vi "PositionerCapture_HoloLoader.vi"() -> ()   [LabVIEW 2011]
doc: "CONEX - CC Virtual Front Panel:\n\nThis is a sample of an application that can be built with the LabVIEW drivers.\n\nPress HOME / ENABLE in top left of panel to put stage in Ready state for motion."
uses:
  <vilib>/userDefined/High Color/IMAQdx.ctl
  C:/Users/Lab541/Desktop/David_Maluenda MAIN FOLDER/System/SupportFiles/Control 1.ctl
  <vilib>/Platform/TimedLoop/XDataNode/timing_clust.ctl
  <vilib>/Platform/TimedLoop/XDataNode/nitl_modes.ctl
  <vilib>/Platform/TimedLoop/XDataNode/wakeup.ctl
  <vilib>/Platform/TimedLoop/XDataNode/XDataNode.xnode
  <vilib>/Platform/TimedLoop/XDataNode/XDNodeRunTimeDep.lvlib
  <vilib>/vision/driver/NI_Vision_Acquisition_Software.lvlib
  <vilib>/vision/NI_Vision_Development_Module.lvlib
panel:
  in  "Units":T1 caption="nm" items=["mm", "um", "nm", "lam"]
  out "test":path
  in  "Session In":T2="BW14bits Paraxial"
  in  "stop":bool
  out "Slide":u8(slide) scale=0.0..100.0
  out "# Sat. Pixels":sgl(slide) scale=1.0..800000.0
  out "Unsatured":bool
  out "pathY":path
  out "pathX":path
  in  "Xoffset1 2":dbl=-1300.0
  out "X position 3":dbl
  in  "Fine: 3":dbl(slide)=8.165680473372781 scale=0.0..10.0
  in  "X position 2":dbl(slide)=3.78698224852071 scale=0.0..10.0
  in  "Yoffset1 2":dbl=-150.0
  out "Y position 2":dbl
  in  "Fine:":dbl(slide)=1.694915254237288 scale=0.0..10.0
  in  "Y position 2":dbl(slide)=1.9318181818181817 scale=0.0..10.0
  in  "Yoffset1":dbl=-300.0
  in  "Xoffset1":dbl=1300.0
  out "Y position 1":dbl
  out "X position":dbl
  in  "Fine:":dbl(slide)=3.8983050847457625 scale=0.0..10.0
  in  "Fine:":dbl(slide)=5.502958579881657 scale=0.0..10.0
  in  "Y position":dbl(slide)=3.5028248587570623 scale=0.0..10.0
  in  "X position 1":dbl(slide)=3.4319526627218933 scale=0.0..10.0
  out "String 4":string
  out "CGHy":T3(plugin-control)
  out "CGHx":T3(plugin-control)
  out "path":path
  in  "Holo:":dbl=1.0
  out "Current noUnits":dbl caption="mm" format="%#_6f"
  in  "lambda":dbl caption="nm" format="%#_6f"
  in  "Units":string(combo)="mm"
  in  "Go0":bool
  in  "Zero position":dbl caption="lam" format="%#_6f"
  in  "Tare":bool
  out "Relative position":dbl caption="lam" format="%#_6f"
  in  "Path to save the captures":path
  out "Image":T3(plugin-control)
  in  "(1) Go to:":dbl=1.0 caption="lam"
  out "Title":string
  in  "Set Max":bool
  in  "Set Min":bool
  in  "Max":dbl
  in  "Min":dbl
  in  "Set velocity":bool
  out "Stop cycle":bool=TRUE
  out "Title 2":string
  in  "Cycle":bool
  in  "Go2":bool
  in  "Go1":bool
  in  "(2) Go to:":dbl=1.0 caption="lam"
  in  "-":bool
  in  "+":bool
  in  "Step:":dbl caption="lam" format="%#_6f"
  out "Position History":dbl(graph)=1.5
  in  "Action":bool
  out "Stop polling":bool=TRUE
  out "Controller state description":string="STATUS"
  out "Velocity MAX":dbl=0.4
  out "Controller state":string="33"
  out "Positioner error":string="0000"
  in  "Velocity:":dbl format="%#_6f"
  in  "Exit":bool=TRUE
  out "Target position":dbl
  in  "Exit":bool
  in  "Position glissière":cluster{dbl, dbl}(slide) scale=0.0..25.0
  out "Current position":dbl caption="lam" format="%#_6f"
  # "mm/s"
  # "mm"
  # "Limits:"
  # "mm"
  # "(1)"
  # "(2)"
  # "%"
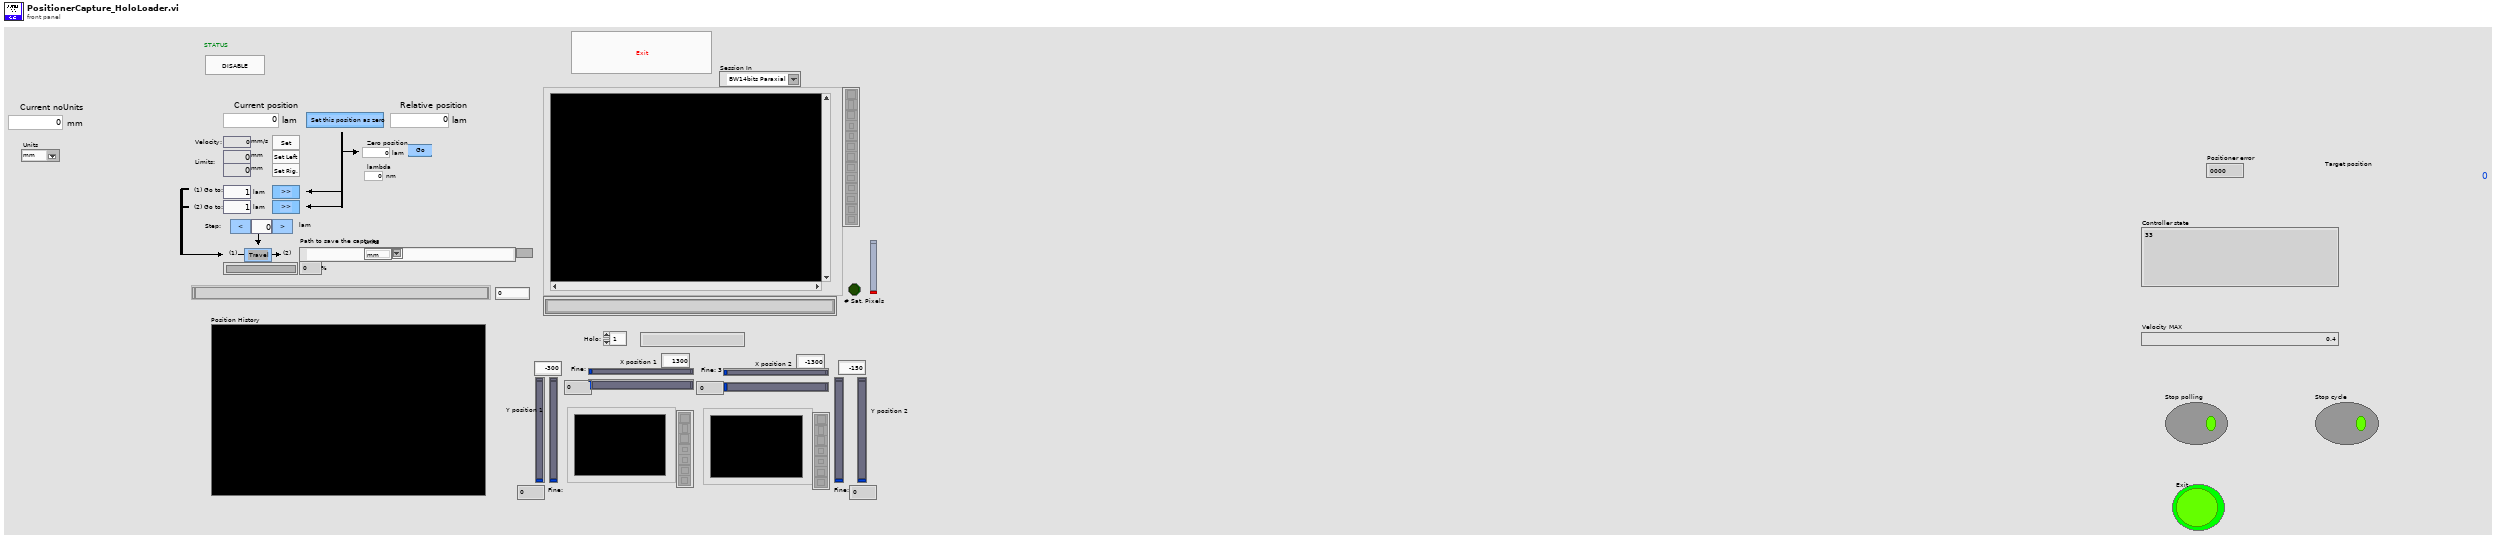
[diagram p1: front panel]
types:
  T1 = typedef "Control 1.ctl" = dbl
  T2 = typedef "IMAQdx.ctl" = refnum<k21>
  T3 = typedef "IMAQ Image.ctl" = refnum<image>
  T4 = enum8{"Enabled", "Disabled", "Disabled and Grayed Out"}
  T5 = typedef "XDNodeRunTimeDep.lvlib/timing_clust.ctl" = cluster{"Expected End [f-1]":u64, "Actual End [f-1]":u64, "Finished Late? [f-1]":bool, "Expected End [i-1]":u64, "Actual End [i-1]":u64, "Finished Late? [i-1]":bool, "Expected Start [i]":u64, "Actual Start [i]":u64, "Expected Start [f]":u64, "Actual Start [f]":u64, "Source Name":string, "Structure Name":string, "Period":i64, "Deadline":i64, "Offset":i64, "Start":i64, "Priority":i32, "Timeout":i32, "Mode":T6, "Wakeup Reason":T7, "Error":errorcluster, "Source Type":string, "Secondary Source Type":string, "Global End Time":u64, "Global Start Time":u64, "Frame Duration":u64, "Iteration Duration":u64, "Assigned CPU":i32, "I/O Scan Engine Mode":u32}
  T6 = typedef "XDNodeRunTimeDep.lvlib/nitl_modes.ctl" = enum32{"No Change", "Process missed periods, maintain original phase", "Discard missed periods, maintain original phase", "Process missed periods, ignore original phase", "Discard missed periods, ignore original phase"}
  T7 = typedef "XDNodeRunTimeDep.lvlib/wakeup.ctl" = enum32{"Normal", "Aborted", "Asynchronous wakeup", "Timing source error", "Timed loop error", "Timeout"}
  T8 = cluster{"VISA resource name":refnum<visa-resource-name>, "Device name":string, "Controller address":i32, "error":errorcluster}
  T9 = cluster{"Starting Value":sgl, "Incremental Value":sgl, "Histogram":u32[]}
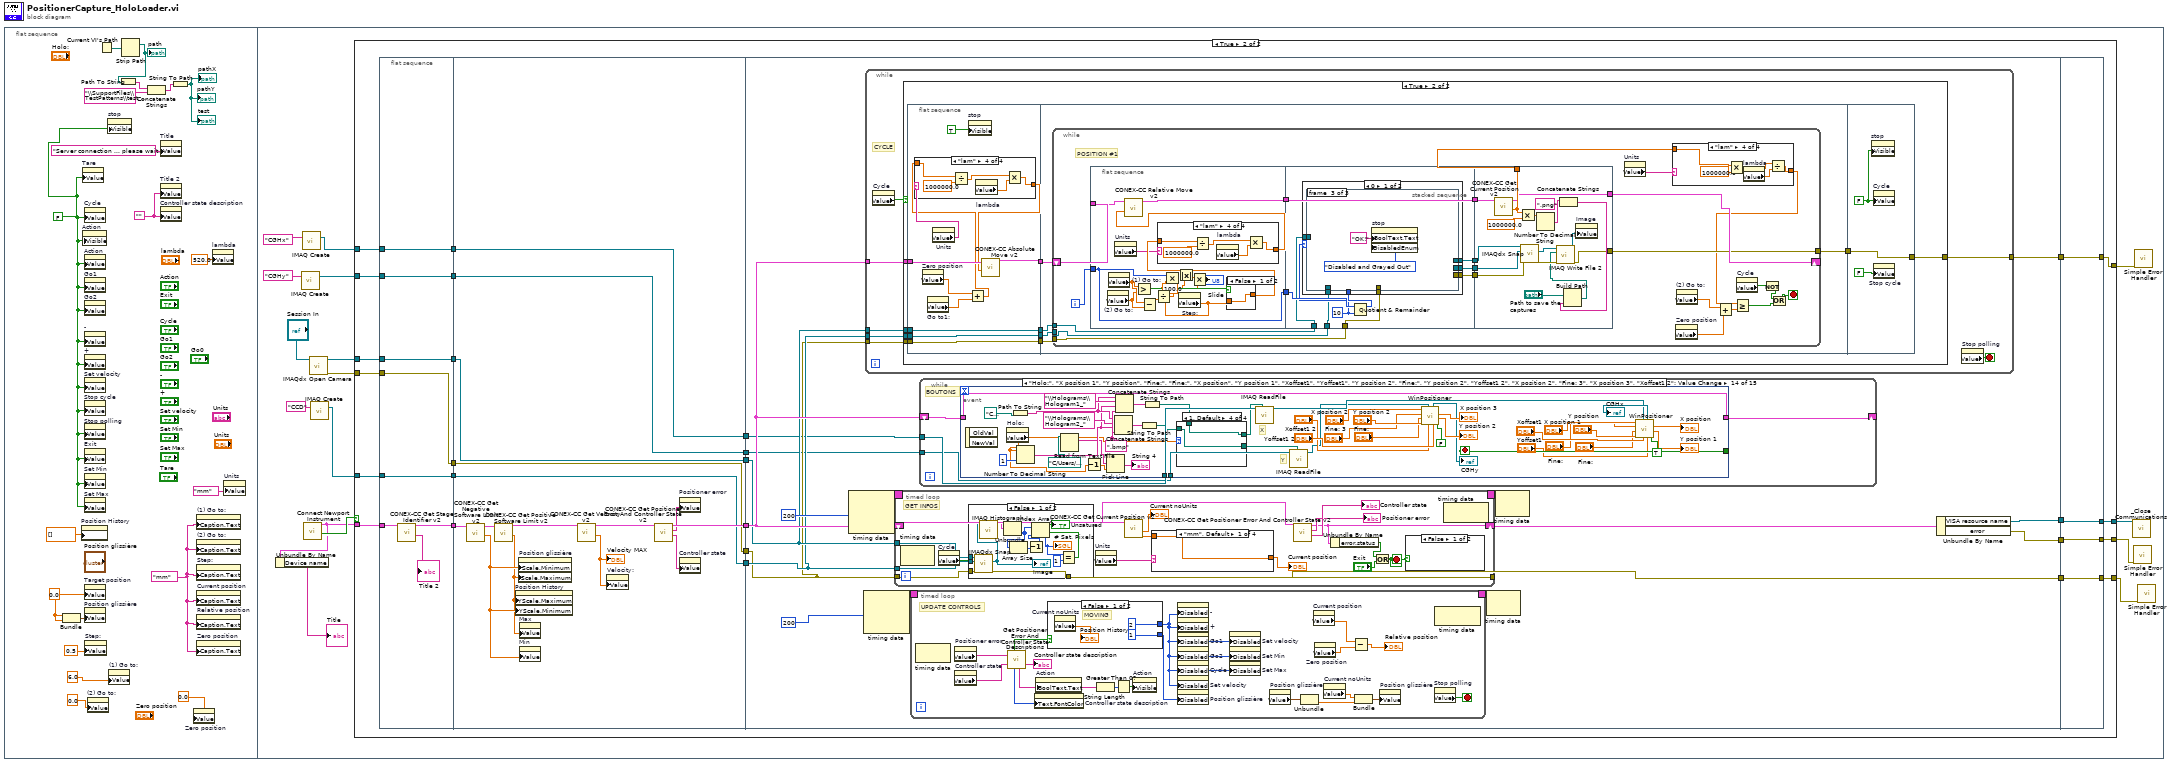
[diagram p0: block diagram]
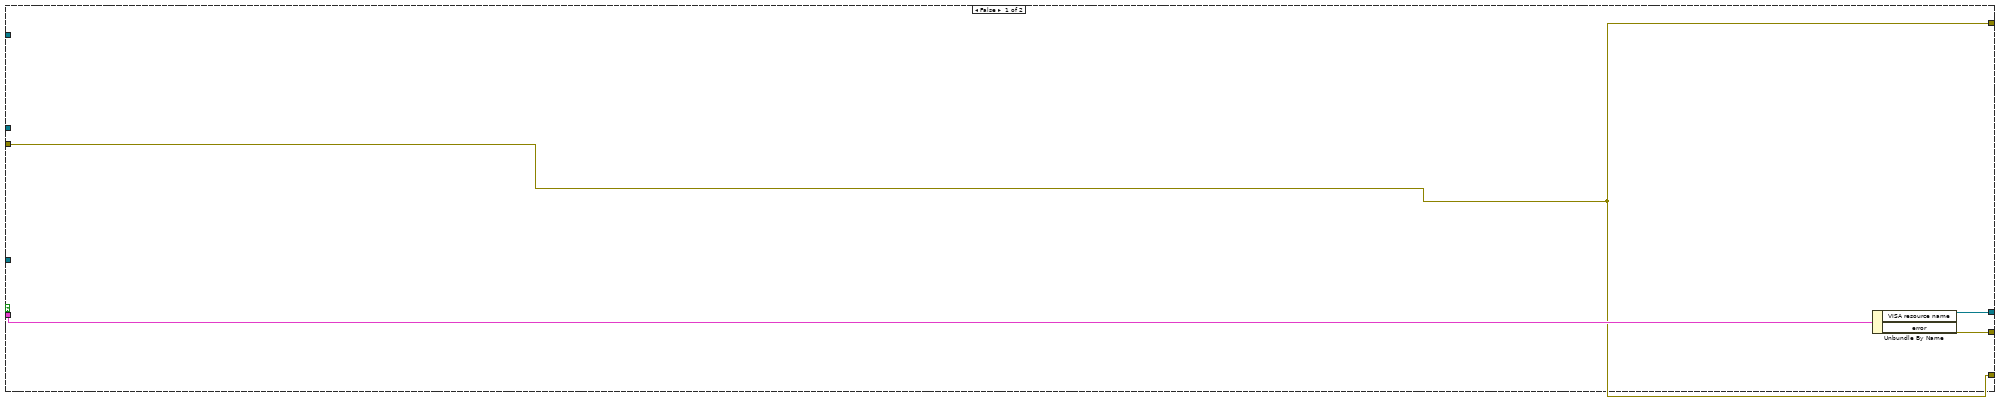
[diagram p2: hidden frame]
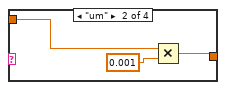
[diagram p5: hidden frame]
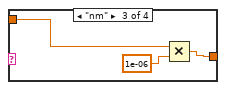
[diagram p6: hidden frame]
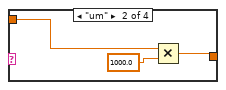
[diagram p8: hidden frame]
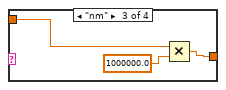
[diagram p9: hidden frame]
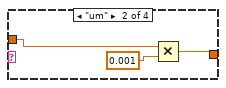
[diagram p11: hidden frame]
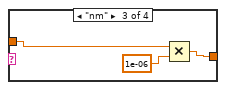
[diagram p12: hidden frame]
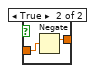
[diagram p13: hidden frame]
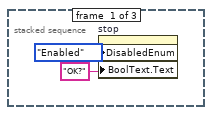
[diagram p14: hidden frame]
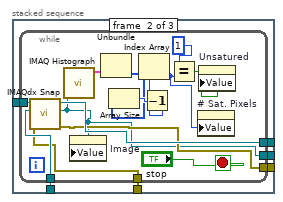
[diagram p15: hidden frame]
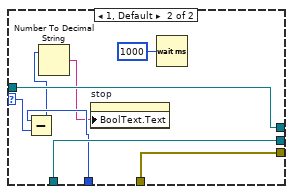
[diagram p16: hidden frame]
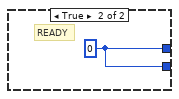
[diagram p17: hidden frame]
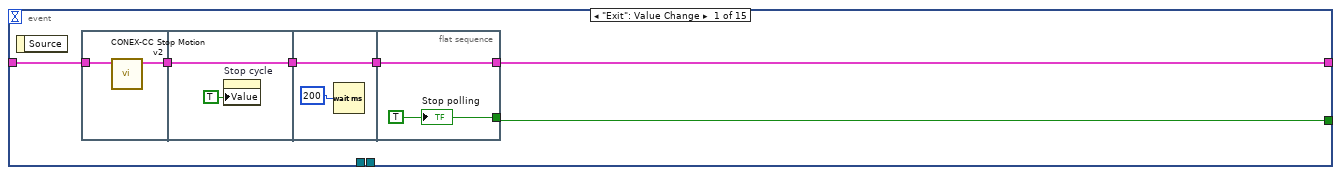
[diagram p18: hidden frame]
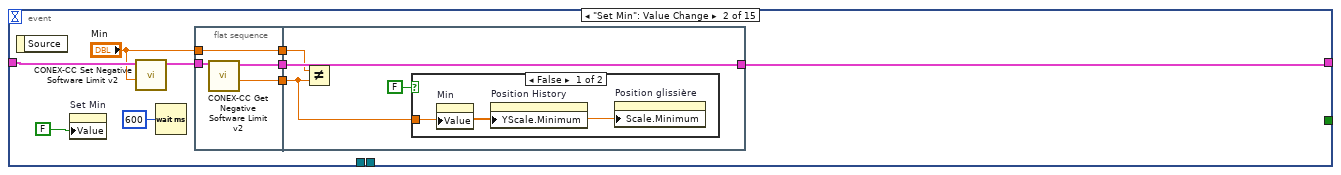
[diagram p19: hidden frame]
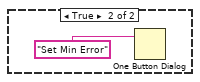
[diagram p20: hidden frame]
diagram:
  n1 = flat-sequence {
    frame #0 {
      w9 = "mm" ("Units")
      w1 = FALSE
      w18 = 0.0
      w17 = ""
      n2 = Bundle(w18, w18) -> (w19:cluster{dbl, dbl})  [unwired: 1 out]
      n3 = property on="Position History" class="WFChart (strict)"("History Data"=dbl[] [] ("Données d'historique")) -> ()  [unwired: 2 in, 2 out]
      n4 = property on="Tare" class="Bool (strict)"("Value"=w1) -> ()  [unwired: 2 in, 2 out]
      n5 = property on="Action" class="Bool (strict)"("Visible"=w1) -> ()  [unwired: 2 in, 2 out]
      n6 = property on="Cycle" class="Bool (strict)"("Value"=w1) -> ()  [unwired: 2 in, 2 out]
      n7 = property on="Action" class="Bool (strict)"("Value"=w1) -> ()  [unwired: 2 in, 2 out]
      n8 = property on="Go1" class="Bool (strict)"("Value"=w1) -> ()  [unwired: 2 in, 2 out]
      n9 = property on="Go2" class="Bool (strict)"("Value"=w1) -> ()  [unwired: 2 in, 2 out]
      n10 = property on="-" class="Bool (strict)"("Value"=w1) -> ()  [unwired: 2 in, 2 out]
      n11 = property on="+" class="Bool (strict)"("Value"=w1) -> ()  [unwired: 2 in, 2 out]
      n12 = property on="Set velocity" class="Bool (strict)"("Value"=w1) -> ()  [unwired: 2 in, 2 out]
      n13 = property on="Stop cycle" class="Bool (strict)"("Value"=w1) -> ()  [unwired: 2 in, 2 out]
      n14 = property on="Stop polling" class="Bool (strict)"("Value"=w1) -> ()  [unwired: 2 in, 2 out]
      n15 = property on="Exit" class="Bool (strict)"("Value"=w1) -> ()  [unwired: 2 in, 2 out]
      n16 = property on="Set Min" class="Bool (strict)"("Value"=w1) -> ()  [unwired: 2 in, 2 out]
      n17 = property on="Set Max" class="Bool (strict)"("Value"=w1) -> ()  [unwired: 2 in, 2 out]
      n18 = property on="Target position" class="DigNum (strict)"("Value"=w18) -> ()  [unwired: 2 in, 2 out]
      n19 = property on="Position glissière" class="Slide (strict)"("Value"=w19) -> ()  [unwired: 2 in, 2 out]
      n20 = property on="Step:" class="DigNum (strict)"("Value"=0.5 ("Step")) -> ()  [unwired: 2 in, 2 out]
      n21 = property on="(2) Go to:" class="DigNum (strict)"("Value"=0.0 ("Abs. Move 2")) -> ()  [unwired: 2 in, 2 out]
      n22 = Current VI's Path() -> (path=w7:path)
      n23 = property on="stop" class="Bool"("Visible"=w1) -> ()  [unwired: 2 in, 2 out]
      n24 = property on="(1) Go to:" class="DigNum (strict)"("Value"=6.0 ("Abs. Move 1")) -> ()  [unwired: 2 in, 2 out]
      n25 = Strip Path(path=w7) -> (stripped path=w6:path)  [unwired: 1 out]
      "path" <- w6
      n26 = Path To String(path=w6) -> (string=w5:string)
      n27 = Concatenate Strings(w5, "\\SupportFiles\\TestPatterns\\test_pattern.bmp" ("string")) -> (w3:string)
      n28 = property on="Title" class="Str"("Value"="Server connection ... please wait." ("Title")) -> ()  [unwired: 2 in, 2 out]
      n29 = property on="Title 2" class="Str"("Value"=w17) -> ()  [unwired: 2 in, 2 out]
      n30 = property on="Controller state description" class="Str"("Value"=w17) -> ()  [unwired: 2 in, 2 out]
      n31 = String To Path(string=w3) -> (path=→"pathX" →"pathY" →"test":path)
      n32 = property on="Zero position" class="DigNum (strict)"("Value"=0.0 ("Zero position")) -> ()  [unwired: 2 in, 2 out]
      n33 = property on="(1) Go to:" class="DigNum (strict)"("Caption.Text"=w9) -> ()  [unwired: 2 in, 2 out]
      n34 = property on="(2) Go to:" class="DigNum (strict)"("Caption.Text"=w9) -> ()  [unwired: 2 in, 2 out]
      n35 = property on="Step:" class="DigNum (strict)"("Caption.Text"=w9) -> ()  [unwired: 2 in, 2 out]
      n36 = property on="Current position" class="DigNum (strict)"("Caption.Text"=w9) -> ()  [unwired: 2 in, 2 out]
      n37 = property on="Relative position" class="DigNum (strict)"("Caption.Text"=w9) -> ()  [unwired: 2 in, 2 out]
      n38 = property on="Zero position" class="DigNum (strict)"("Caption.Text"=w9) -> ()  [unwired: 2 in, 2 out]
      n39 = property on="lambda" class="DigNum (strict)"("Value"=520.0 ("lambda")) -> ()  [unwired: 2 in, 2 out]
      n40 = property on="Units" class="CmbBox"("Value"="mm" ("Units")) -> ()  [unwired: 2 in, 2 out]
    }
    frame #1 {
      n41 = call "IMAQ Create"("Image Name"="CGHy") -> ("New Image"=w21:T3)  [unwired: 4 in, 1 out]
      n42 = call "IMAQ Create"("Image Name"="CGHx") -> ("New Image"=w20:T3)  [unwired: 4 in, 1 out]
      n43 = call <userlib>:"Connect Newport Instrument.vi"() -> ("Connected"=w33:bool, "Device Connection Cluster"=w32:T8)  [unwired: 7 in, 3 out]
      n44 = Unbundle By Name(w32) -> ("Device name"=→"Title":string)
      n45 = call <vilib>:"IMAQdx Open Camera.vi"("Session In"="Session In") -> ("error out"=w26:errorcluster, "Session Out"=w28:T2)  [unwired: 9 in]
      n46 = call "IMAQ Create"("Image Name"="CCD") -> ("New Image"=w27:T3)  [unwired: 4 in, 1 out]
      n47 = case shown="True" w33 {
        tunnel: [w38 w65] -> w35
        tunnel: w32 -> [w39 w63]
        tunnel: [w37 w59] -> w31
        tunnel: w28 -> [_ w57]
        tunnel: w27 -> [_ w54]
        tunnel: w26 -> [w36 w51]
        tunnel: [w36 w48] -> w25
        tunnel: [w36 w46] -> w24
        tunnel: w21 -> [_ w44]
        tunnel: w20 -> [_ w41]
        frame False {
          n48 = Unbundle By Name(w39) -> ("VISA resource name"=w37:refnum<visa-resource-name>, "error"=w38:errorcluster)
        }
        frame True {
          n49 = flat-sequence {
            tunnel: w63 -> [w73]
            tunnel: [w71] -> w62
            tunnel: [w70] -> w58
            tunnel: w57 -> [w70]
            tunnel: [w69] -> w55
            tunnel: w54 -> [w69]
            tunnel: [w68] -> w52
            tunnel: w51 -> [w68]
            tunnel: [w67] -> w45
            tunnel: w44 -> [w67]
            tunnel: [w66] -> w42
            tunnel: w41 -> [w66]
            tunnel: [w85] -> w64
            tunnel: w62 -> [w82]
            tunnel: w58 -> [w78]
            tunnel: [w78] -> w56
            tunnel: w55 -> [w77]
            tunnel: [w77] -> w53
            tunnel: w52 -> [w76]
            tunnel: [w76] -> w50
            tunnel: w45 -> [w75]
            tunnel: [w75] -> w43
            tunnel: w42 -> [w74]
            tunnel: [w74] -> w40
            tunnel: w64 -> [w96]
            tunnel: [w98] -> w61
            tunnel: [w97] -> w60
            tunnel: w56 -> [w95]
            tunnel: w53 -> [w94]
            tunnel: w50 -> [w93]
            tunnel: [w92] -> w49
            tunnel: [w91] -> w47
            tunnel: w43 -> [w90]
            tunnel: w40 -> [w89]
            tunnel: [w616] -> w65
            tunnel: w61 -> [w615]
            tunnel: w60 -> [w616]
            tunnel: [w615] -> w59
            tunnel: [w614] -> w48
            tunnel: w49 -> [w614]
            tunnel: [w613] -> w46
            tunnel: w47 -> [w613]
            frame #0 {
              n50 = call <userlib>:"CONEX-CC Get Stage Identifier v2.vi"("Connection Cluster in"=w73) -> ("Identifier"=→"Title 2":string, "Connection Cluster out"=w71:T8)  [unwired: 9 in]
            }
            frame #1 {
              n51 = call <userlib>:"CONEX-CC Get Negative Software Limit v2.vi"("Connection Cluster in"=w82) -> ("Left limit"=w87:dbl, "Connection Cluster out"=w81:T8)  [unwired: 9 in]
              n52 = call <userlib>:"CONEX-CC Get Positive Software Limit v2.vi"("Connection Cluster in"=w81) -> ("Right limit"=w86:dbl, "Connection Cluster out"=w80:T8)  [unwired: 9 in]
              n53 = property on="Position History" class="WFChart (strict)"("YScale.Maximum"=w86, "YScale.Minimum"=w87) -> ()  [unwired: 2 in, 2 out]
              n54 = property on="Position glissière" class="Slide (strict)"("Scale.Minimum"=w87, "Scale.Maximum"=w86) -> ()  [unwired: 2 in, 2 out]
              n55 = property on="Max" class="DigNum (strict)"("Value"=w86) -> ()  [unwired: 2 in, 2 out]
              n56 = property on="Min" class="DigNum (strict)"("Value"=w87) -> ()  [unwired: 2 in, 2 out]
              n57 = call <userlib>:"CONEX-CC Get Velocity v2.vi"("Connection Cluster in"=w80) -> ("Velocity"=w88:dbl, "Connection Cluster out"=w79:T8)  [unwired: 8 in, 1 out]
              "Velocity MAX" <- w88
              n58 = property on="Velocity:" class="DigNum (strict)"("Value"=w88) -> ()  [unwired: 2 in, 2 out]
              n59 = call <userlib>:"CONEX-CC Get Positioner Error And Controller State v2.vi"("Connection Cluster in"=w79) -> ("Controller state"=w83:string, "Positioner error"=w84:string, "Connection Cluster out"=w85:T8)  [unwired: 8 in]
              n60 = property on="Positioner error" class="Str"("Value"=w84) -> ()  [unwired: 2 in, 2 out]
              n61 = property on="Controller state" class="Str"("Value"=w83) -> ()  [unwired: 2 in, 2 out]
            }
            frame #2 {
              n62 = node-c288(i64 200 ("Période")) -> (w105:T5)  [unwired: 1 in, 1 out]
              n63 = node-c288(i64 200 ("Période")) -> (w103:T5)  [unwired: 1 in, 1 out]
              n64 = while {
                tunnel: w96 -> [w112]
                tunnel: w95 -> [w109]
                tunnel: w94 -> [w108]
                tunnel: w93 -> [w107]
                tunnel: [w106] -> w91
                stop <- w111 stop-if-true
                # "CYCLE"
                n65 = property on="Cycle" class="Bool (strict)"() -> ("Value"=w110:bool)  [unwired: 2 in, 2 out]
                n66 = case shown="True" w110 {
                  tunnel: w112 -> [_ w123]
                  tunnel: w109 -> [_ w120]
                  tunnel: w108 -> [_ w118]
                  tunnel: w107 -> [w113 w116]
                  tunnel: [w113 w115] -> w106
                  frame False {
                  }
                  frame True {
                    n67 = flat-sequence {
                      tunnel: w123 -> [w134]
                      tunnel: [w133] -> w122
                      tunnel: [w132] -> w121
                      tunnel: w120 -> [w132]
                      tunnel: [w131] -> w119
                      tunnel: w118 -> [w131]
                      tunnel: [w130] -> w117
                      tunnel: w116 -> [w130]
                      tunnel: w122 -> [w151]
                      tunnel: w121 -> [w150]
                      tunnel: w119 -> [w149]
                      tunnel: w117 -> [w148]
                      tunnel: [w147] -> w114
                      tunnel: [w284] -> w115
                      tunnel: w114 -> [w284]
                      frame #0 {
                        n68 = property on="Zero position" class="DigNum (strict)"() -> ("Value"=w125:dbl)  [unwired: 2 in, 2 out]
                        n69 = property on="Go to1:" class="DigNum (strict)"() -> ("Value"=w127:dbl)  [unwired: 2 in, 2 out]
                        n70 = property on="Units" class="CmbBox"() -> ("Value"=w128:string)  [unwired: 2 in, 2 out]
                        n71 = property on="stop" class="Bool"("Visible"=TRUE) -> ()  [unwired: 2 in, 2 out]
                        n72 = Add(x=w125, y=w127) -> (x+y=w126:dbl)
                        n73 = case shown="\"lam\"" w128 {
                          tunnel: [w135 w136 w139 w142] -> w129
                          tunnel: w126 -> [w135 w137 w140 w146]
                          frame "mm", Default {
                          }
                          frame "um" {
                            n74 = Multiply(x=w137, y=0.001) -> (x*y=w136:dbl)
                          }
                          frame "nm" {
                            n75 = Multiply(x=w140, y=1e-06) -> (x*y=w139:dbl)
                          }
                          frame "lam" {
                            n76 = Divide(x=w146, y=1000000.0) -> (x/y=w144:dbl)
                            n77 = property on="lambda" class="DigNum (strict)"() -> ("Value"=w143:dbl)  [unwired: 2 in, 2 out]
                            n78 = Multiply(x=w144, y=w143) -> (x*y=w142:dbl)
                          }
                        }
                        n79 = call <userlib>:"CONEX-CC Absolute Move v2.vi"("Target position"=w129, "Connection Cluster in"=w134) -> ("Connection Cluster out"=w133:T8)  [unwired: 5 in, 2 out]
                      }
                      frame #1 {
                        n80 = while {
                          shift-right: [w173] -> _
                          shift-left: w151 -> [w174]
                          tunnel: w150 -> [w163]
                          tunnel: w149 -> [w162]
                          tunnel: w148 -> [w161]
                          tunnel: [w172] -> w147
                          i -> [w160]
                          stop <- w159 stop-if-true
                          # "POSITION #1"
                          n81 = flat-sequence {
                            tunnel: w174 -> [w202]
                            tunnel: [w201] -> w166
                            tunnel: w160 -> [w187]
                            tunnel: [w187] -> w155
                            tunnel: w166 -> [w227]
                            tunnel: [w227] -> w165
                            tunnel: w163 -> [w224]
                            tunnel: w162 -> [w223]
                            tunnel: w161 -> [w222]
                            tunnel: w155 -> [w226]
                            tunnel: [w221] -> w154
                            tunnel: [w220] -> w153
                            tunnel: [w219] -> w152
                            tunnel: w165 -> [w279]
                            tunnel: [w271] -> w171
                            tunnel: [w270] -> w173
                            tunnel: [w269] -> w172
                            tunnel: w154 -> [w268]
                            tunnel: w153 -> [w267]
                            tunnel: w152 -> [w266]
                            frame #0 {
                              n82 = property on="(2) Go to:" class="DigNum (strict)"() -> ("Value"=w194:dbl)  [unwired: 2 in, 2 out]
                              n83 = property on="(1) Go to:" class="DigNum (strict)"() -> ("Value"=w195:dbl)  [unwired: 2 in, 2 out]
                              n84 = property on="Units" class="CmbBox"() -> ("Value"=w197:string)  [unwired: 2 in, 2 out]
                              n85 = Greater?(x=w195, y=w194) -> (0:w200:bool)
                              n86 = Subtract(x=w195, y=w194) -> (x-y=w192:dbl)
                              n87 = property on="Step:" class="DigNum (strict)"() -> ("Value"=w196:dbl)  [unwired: 2 in, 2 out]
                              n88 = Multiply(x=w187, y=w196) -> (x*y=w193:dbl)
                              n89 = Divide(x=w193, y=w192) -> (x/y=w191:dbl)
                              n90 = Absolute Value(x=w191) -> (abs(x)=w190:dbl)
                              n91 = Multiply(x=w190, y=100.0) -> (x*y=→"Slide":dbl)
                              n92 = case shown="False" w200 {
                                tunnel: [w215 w216] -> w199
                                tunnel: w196 -> [w215 w217]
                                frame False {
                                }
                                frame True {
                                n93 = Negate(x=w217) -> (-x=w216:dbl)
                                }
                              }
                              n94 = case shown="\"lam\"" w197 {
                                tunnel: [w203 w205 w208 w211] -> w198
                                tunnel: w199 -> [w203 w204 w207 w210]
                                frame "mm", Default {
                                }
                                frame "um" {
                                n95 = Multiply(x=w204, y=0.001) -> (x*y=w205:dbl)
                                }
                                frame "nm" {
                                n96 = Multiply(x=w207, y=1e-06) -> (x*y=w208:dbl)
                                }
                                frame "lam" {
                                n97 = Divide(x=w210, y=1000000.0) -> (x/y=w213:dbl)
                                n98 = property on="lambda" class="DigNum (strict)"() -> ("Value"=w212:dbl)  [unwired: 2 in, 2 out]
                                n99 = Multiply(x=w213, y=w212) -> (x*y=w211:dbl)
                                }
                              }
                              n100 = call <userlib>:"CONEX-CC Relative Move v2.vi"("Relative displacement"=w198, "Connection Cluster in"=w202) -> ("Connection Cluster out"=w201:T8)  [unwired: 9 in]
                            }
                            frame #1 {
                              w218 = 10 ("y")
                              n101 = Quotient & Remainder(x=w226, y=w218) -> (x-y*floor(x/y)=w225:i32)  [unwired: 1 out]
                              n102 = case shown="0" w225 {
                                selector: w225 -> [_ w261]
                                tunnel: w224 -> [w233 w265]
                                tunnel: w223 -> [w232 w264]
                                tunnel: w222 -> [w231 w263]
                                tunnel: [w230 w265] -> w221
                                tunnel: [w229 w264] -> w220
                                tunnel: [w228 w263] -> w219
                                tunnel: w218 -> [_ w260]
                                frame 0 {
                                n103 = stacked-sequence {
                                tunnel: w233 -> [_ w241 _]
                                tunnel: w232 -> [_ w240 _]
                                tunnel: w231 -> [_ w239 _]
                                tunnel: [_ w238 _] -> w230
                                tunnel: [_ w237 _] -> w229
                                tunnel: [_ w236 _] -> w228
                                frame #0 {
                                n104 = property on="stop" class="Bool"("DisabledEnum"=T4."Enabled" ("Disabled"), "BoolText.Text"="OK?" ("Boolean Text.Text")) -> ()  [unwired: 2 in, 2 out]
                                }
                                frame #1 {
                                n105 = while {
                                tunnel: w241 -> [w247]
                                tunnel: w240 -> [w246]
                                tunnel: w239 -> [w245]
                                tunnel: [w244] -> w238
                                tunnel: [w242] -> w237
                                tunnel: [w243] -> w236
                                stop <- "stop" stop-if-true
                                n106 = call <vilib>:"IMAQdx Snap.vi"("error in"=w245, "Image In"=w246, "Session In"=w247) -> ("error out"=w243:errorcluster, "Image Out"=w242:T3, "Session Out"=w244:T2)  [unwired: 6 in]
                                n107 = call "IMAQ Histograph"("Image"=w242) -> ("Histogram Graph"=w249:T9)  [unwired: 7 in, 3 out]
                                n108 = property on="Image" class="ImageControl"("Value"=w242) -> ()  [unwired: 2 in, 2 out]
                                n109 = Unbundle(w249) -> ("Histogram"=w250:u32[])  [unwired: 2 out]
                                n110 = Array Size(array=w250) -> (size(s)=w251:i32)
                                n111 = Decrement(x=w251) -> (x-1=w252:i32)
                                n112 = Index Array(array=w250, index=w252) -> (element=w254:u32)
                                n113 = Equal?(x=u32 1 ("y"), y=w254) -> (x = y?=w255:bool)
                                n114 = property on="# Sat. Pixels" class="Slide (strict)"("Value"=w254) -> ()  [unwired: 2 in, 2 out]
                                n115 = property on="Unsatured" class="Bool"("Value"=w255) -> ()  [unwired: 2 in, 2 out]
                                }
                                }
                                frame #2 {
                                n116 = property on="stop" class="Bool"("BoolText.Text"="OK!" ("Boolean Text.Text"), "DisabledEnum"=T4."Disabled and Grayed Out" ("Disabled")) -> ()  [unwired: 2 in, 2 out]
                                }
                                }
                                }
                                frame 1, Default {
                                n117 = Subtract(x=w260, y=w261) -> (x-y=w259:i32)
                                n118 = Number To Decimal String(number=w259) -> (decimal integer string=w258:string)  [unwired: 1 in]
                                n119 = property on="stop" class="Bool"("BoolText.Text"=w258) -> ()  [unwired: 2 in, 2 out]
                                n120 = Wait (ms)(milliseconds to wait=u32 1000) -> ()  [unwired: 1 out]
                                }
                              }
                            }
                            frame #2 {
                              n121 = call <userlib>:"CONEX-CC Get Current Position v2.vi"("Connection Cluster in"=w279) -> ("Current position"=w271:dbl, "Connection Cluster out"=w270:T8)  [unwired: 8 in, 1 out]
                              n122 = Multiply(x=w271, y=1000000.0) -> (x*y=w275:dbl)
                              n123 = call <vilib>:"IMAQdx Snap.vi"("error in"=w266, "Image In"=w267, "Session In"=w268) -> ("error out"=w281:errorcluster, "Image Out"=w282:T3)  [unwired: 6 in, 1 out]
                              n124 = Number To Decimal String(number=w275) -> (decimal integer string=w274:string)  [unwired: 1 in]
                              n125 = Concatenate Strings(w274, ".png" ("string")) -> (w272:string)
                              n126 = Build Path(base path="Path to save the captures", name or relative path=w272) -> (appended path=w276:path)
                              n127 = call-poly "IMAQ Write File 2"("error in (no error)"=w281, "File Path"=w276, "Image"=w282) -> ("error out"=w269:errorcluster, "Image Out (duplicate)"=w280:T3)  [unwired: 7 in]
                              n128 = property on="Image" class="ImageControl"("Value"=w280) -> ()  [unwired: 2 in, 2 out]
                            }
                          }
                          n129 = property on="Units" class="CmbBox"() -> ("Value"=w164:string)  [unwired: 2 in, 2 out]
                          n130 = case shown="\"lam\"" w164 {
                            tunnel: [w175 w176 w179 w182] -> w170
                            tunnel: w171 -> [w175 w177 w180 w183]
                            frame "mm", Default {
                            }
                            frame "um" {
                              n131 = Multiply(x=w177, y=1000.0) -> (x*y=w176:dbl)
                            }
                            frame "nm" {
                              n132 = Multiply(x=w180, y=1000000.0) -> (x*y=w179:dbl)
                            }
                            frame "lam" {
                              n133 = Multiply(x=w183, y=1000000.0) -> (x*y=w186:dbl)
                              n134 = property on="lambda" class="DigNum (strict)"() -> ("Value"=w184:dbl)  [unwired: 2 in, 2 out]
                              n135 = Divide(x=w186, y=w184) -> (x/y=w182:dbl)
                            }
                          }
                          n136 = property on="Zero position" class="DigNum (strict)"() -> ("Value"=w167:dbl)  [unwired: 2 in, 2 out]
                          n137 = property on="(2) Go to:" class="DigNum (strict)"() -> ("Value"=w168:dbl)  [unwired: 2 in, 2 out]
                          n138 = Add(x=w168, y=w167) -> (x+y=w169:dbl)
                          n139 = Greater Or Equal?(x=w170, y=w169) -> (x >= y?=w158:bool)
                          n140 = property on="Cycle" class="Bool (strict)"() -> ("Value"=w156:bool)  [unwired: 2 in, 2 out]
                          n141 = Not(x=w156) -> (.not. x?=w157:bool)
                          n142 = Or(x=w157, y=w158) -> (x .or. y?=w159:bool)
                        }
                      }
                      frame #2 {
                        w283 = FALSE ("Cycle")
                        n143 = property on="stop" class="Bool"("Visible"=w283) -> ()  [unwired: 2 in, 2 out]
                        n144 = property on="Cycle" class="Bool (strict)"("Value"=w283) -> ()  [unwired: 2 in, 2 out]
                        n145 = property on="Stop cycle" class="Bool (strict)"("Value"=FALSE ("Cycle")) -> ()  [unwired: 2 in, 2 out]
                      }
                    }
                  }
                }
                n146 = property on="Stop polling" class="Bool (strict)"() -> ("Value"=w111:bool)  [unwired: 2 in, 2 out]
              }
              n147 = timed-loop {
                timing: w105 -> [_]
                timing-out: [_] -> w104
                shift-right: [w570] -> w99
                shift-left: w96 -> [w580]
                tunnel: w95 -> [w579]
                tunnel: w94 -> [w578]
                tunnel: w93 -> [w577]
                tunnel: [w576] -> w92
                stop <- w573 stop-if-true
                # "GET INFOS"
                n148 = node-c288() -> ()  [unwired: 2 out]
                n149 = property on="Cycle" class="Bool (strict)"() -> ("Value"=w575:bool)  [unwired: 2 in, 2 out]
                n150 = case shown="False" w575 {
                  tunnel: w579 -> [w604 _]
                  tunnel: w578 -> [w603 _]
                  tunnel: w577 -> [w602 w605]
                  tunnel: [w601 w605] -> w576
                  frame False {
                    n151 = call <vilib>:"IMAQdx Snap.vi"("error in"=w602, "Image In"=w603, "Session In"=w604) -> ("error out"=w601:errorcluster, "Image Out"=w600:T3)  [unwired: 6 in, 1 out]
                    "Image" <- w600
                    n152 = call "IMAQ Histograph"("Image"=w600) -> ("Histogram Graph"=w599:T9)  [unwired: 7 in, 3 out]
                    n153 = Unbundle(w599) -> ("Histogram"=w597:u32[])  [unwired: 2 out]
                    n154 = Array Size(array=w597) -> (size(s)=w598:i32)
                    n155 = Decrement(x=w598) -> (x-1=w596:i32)
                    n156 = Index Array(array=w597, index=w596) -> (element=w593:u32)
                    "# Sat. Pixels" <- w593
                    n157 = Equal?(x=w593, y=u32 1) -> (x = y?=→"Unsatured":bool)
                  }
                  frame True {
                  }
                }
                n158 = property on="Units" class="CmbBox"() -> ("Value"=w565:string)  [unwired: 2 in, 2 out]
                n159 = call <userlib>:"CONEX-CC Get Current Position v2.vi"("Connection Cluster in"=w580) -> ("Current position"=w566:dbl, "Connection Cluster out"=w567:T8)  [unwired: 8 in, 1 out]
                "Current noUnits" <- w566
                n160 = case shown="\"mm\", Default" w565 {
                  tunnel: [w581 w582 w585 w588] -> w569
                  tunnel: w566 -> [w581 w583 w586 w589]
                  frame "mm", Default {
                  }
                  frame "um" {
                    n161 = Multiply(x=w583, y=1000.0) -> (x*y=w582:dbl)
                  }
                  frame "nm" {
                    n162 = Multiply(x=w586, y=1000000.0) -> (x*y=w585:dbl)
                  }
                  frame "lam" {
                    n163 = Multiply(x=w589, y=1000000.0) -> (x*y=w592:dbl)
                    n164 = property on="lambda" class="DigNum (strict)"() -> ("Value"=w590:dbl)  [unwired: 2 in, 2 out]
                    n165 = Divide(x=w592, y=w590) -> (x/y=w588:dbl)
                  }
                }
                "Current position" <- w569
                n166 = call <userlib>:"CONEX-CC Get Positioner Error And Controller State v2.vi"("Connection Cluster in"=w567) -> ("Controller state"=→"Controller state":string, "Positioner error"=→"Positioner error":string, "Connection Cluster out"=w570:T8)  [unwired: 8 in]
                n167 = Unbundle By Name(w570) -> ("error.status"=w568:bool)
                n168 = Or(x=w568, y="Exit") -> (x .or. y?=w573:bool)
                n169 = case shown="False" w573 {
                  frame False {
                  }
                  frame True {
                    n170 = property on="Exit" class="Bool (strict)"("Val(Sgnl)"=TRUE) -> ()  [unwired: 2 in, 2 out]
                  }
                }
                n171 = node-c288() -> ()  [unwired: 2 out]
              }
              n172 = timed-loop {
                timing: w103 -> [_]
                timing-out: [_] -> w102
                stop <- w294 stop-if-true
                # "UPDATE CONTROLS"
                n173 = node-c288() -> ()  [unwired: 2 out]
                n174 = property on="Positioner error" class="Str"() -> ("Value"=w303:string)  [unwired: 2 in, 2 out]
                n175 = property on="Controller state" class="Str"() -> ("Value"=w302:string)  [unwired: 2 in, 2 out]
                n176 = call <userlib>:"Get Positioner Error And Controller State Descriptions.vi"("Controller state"=w302, "Positioner error"=w303) -> ("Color"=w300:u32, "Action name"=w299:string, "Controller state description"=→"Controller state description":string, "IsReady?"=w296:bool)  [unwired: 2 out]
                n177 = property on="Controller state description" class="Str"("Text.FontColor"=w300) -> ()  [unwired: 2 in, 2 out]
                n178 = property on="Action" class="Bool (strict)"("BoolText.Text"=w299) -> ()  [unwired: 2 in, 2 out]
                n179 = case shown="False" w296 {
                  tunnel: [u8 2 w307] -> w293
                  tunnel: [u8 1 w307] -> w295
                  frame False {
                    # "MOVING"
                    n180 = property on="Current noUnits" class="DigNum (strict)"() -> ("Value"=→"Position History":dbl)  [unwired: 2 in, 2 out]
                  }
                  frame True {
                    w307 = u8 0
                    # "READY"
                  }
                }
                n181 = String Length(string=w299) -> (length=w298:i32)
                n182 = Greater Than 0?(x=w298) -> (x > 0?=w297:bool)
                n183 = property on="Action" class="Bool (strict)"("Visible"=w297) -> ()  [unwired: 2 in, 2 out]
                n184 = property on="-" class="Bool (strict)"("Disabled"=w293) -> ()  [unwired: 2 in, 2 out]
                n185 = property on="+" class="Bool (strict)"("Disabled"=w293) -> ()  [unwired: 2 in, 2 out]
                n186 = property on="Go1" class="Bool (strict)"("Disabled"=w293) -> ()  [unwired: 2 in, 2 out]
                n187 = property on="Go2" class="Bool (strict)"("Disabled"=w293) -> ()  [unwired: 2 in, 2 out]
                n188 = property on="Cycle" class="Bool (strict)"("Disabled"=w293) -> ()  [unwired: 2 in, 2 out]
                n189 = property on="Set velocity" class="Bool (strict)"("Disabled"=w293) -> ()  [unwired: 2 in, 2 out]
                n190 = property on="Position glissière" class="Slide (strict)"("Disabled"=w295) -> ()  [unwired: 2 in, 2 out]
                n191 = property on="Set velocity" class="Bool (strict)"("Disabled"=w293) -> ()  [unwired: 2 in, 2 out]
                n192 = property on="Set Min" class="Bool (strict)"("Disabled"=w293) -> ()  [unwired: 2 in, 2 out]
                n193 = property on="Set Max" class="Bool (strict)"("Disabled"=w293) -> ()  [unwired: 2 in, 2 out]
                n194 = property on="Position glissière" class="Slide (strict)"() -> ("Value"=w291:cluster{dbl, dbl})  [unwired: 2 in, 2 out]
                n195 = Unbundle(w291) -> (w290:dbl)  [unwired: 1 out]
                n196 = property on="Current position" class="DigNum (strict)"() -> ("Value"=w286:dbl)  [unwired: 2 in, 2 out]
                n197 = property on="Zero position" class="DigNum (strict)"() -> ("Value"=w287:dbl)  [unwired: 2 in, 2 out]
                n198 = property on="Current noUnits" class="DigNum (strict)"() -> ("Value"=w288:dbl)  [unwired: 2 in, 2 out]
                n199 = Subtract(x=w286, y=w287) -> (x-y=→"Relative position":dbl)
                n200 = Bundle("Value"=w288, w290) -> (w292:cluster{"Value":dbl, dbl})  [unwired: 1 out]
                n201 = property on="Position glissière" class="Slide (strict)"("Value"=w292) -> ()  [unwired: 2 in, 2 out]
                n202 = node-c288() -> ()  [unwired: 2 out]
                n203 = property on="Stop polling" class="Bool (strict)"() -> ("Value"=w294:bool)  [unwired: 2 in, 2 out]
              }
              n204 = while {
                shift-right: [w316] -> _
                shift-left: w96 -> [w318]
                tunnel: w90 -> [w314]
                tunnel: w89 -> [w315]
                stop <- w317 stop-if-true
                # "BOUTONS"
                n205 = event shown="[13] \"Holo:\", \"X position 1\", \"Y position\", \"Fine:\", \"Fine:\", \"X position\", \"Y position 1\", \"Xoffset1\", \"Yoffset1\", \"Y position 2\", \"Fine:\", \"Y position 2\", \"Yoffset1 2\", \"X position 2\", \"Fine: 3\", \"X position 3\", \"Xoffset1 2\": Value Change" {
                  selector: _ -> [_ _ _ _ _ _ _ _ _ _ _ _ _ _ _]
                  dyn-events: _ -> [_ _ _ _ _ _ _ _ _ _ _ _ _ _ _]
                  timeout: _ -> [_ _ _ _ _ _ _ _ _ _ _ _ _ _ _]
                  tunnel: [w322 _ _ _ _ _ _ _ _ _ _ _ _ _ _] -> w317
                  tunnel: w318 -> [w319 w339 w353 w366 w378 w382 w401 w422 w443 w463 w480 w496 w498 w530 w556]
                  tunnel: [w324 w338 w352 w363 w377 w381 w400 w423 w442 w462 w481 w496 w498 w530 w556] -> w316
                  tunnel: w315 -> [_ _ _ _ _ _ _ _ _ _ _ _ _ w513 _]
                  tunnel: w314 -> [_ _ _ _ _ _ _ _ _ _ _ _ _ w512 _]
                  event "Exit": Value Change {
                    n206 = event-data() -> ()  [unwired: 2 out]
                    n207 = flat-sequence {
                      tunnel: [w326] -> w323
                      tunnel: w319 -> [w325]
                      tunnel: w323 -> [w328]
                      tunnel: [w328] -> w321
                      tunnel: w321 -> [w330]
                      tunnel: [w330] -> w320
                      tunnel: [w332] -> w324
                      tunnel: w320 -> [w332]
                      tunnel: [w331] -> w322
                      frame #0 {
                        n208 = call <userlib>:"CONEX-CC Stop Motion v2.vi"("Connection Cluster in"=w325) -> ("Connection Cluster out"=w326:T8)  [unwired: 10 in]
                      }
                      frame #1 {
                        n209 = property on="Stop cycle" class="Bool (strict)"("Value"=TRUE) -> ()  [unwired: 2 in, 2 out]
                      }
                      frame #2 {
                        n210 = Wait (ms)(milliseconds to wait=u32 200 ("attente (ms)")) -> ()  [unwired: 1 out]
                      }
                      frame #3 {
                        w331 = TRUE
                        "Stop polling" <- w331
                      }
                    }
                  }
                  event "Set Min": Value Change {
                    n211 = event-data() -> ()  [unwired: 2 out]
                    n212 = property on="Set Min" class="Bool (strict)"("Value"=FALSE ("Set Min")) -> ()  [unwired: 2 in, 2 out]
                    n213 = call <userlib>:"CONEX-CC Set Negative Software Limit v2.vi"("Negative limit (left)"="Min", "Connection Cluster in"=w339) -> ("Connection Cluster out"=w341:T8)  [unwired: 9 in]
                    n214 = Wait (ms)(milliseconds to wait=u32 600 ("attente (ms)")) -> ()  [unwired: 1 out]
                    n215 = flat-sequence {
                      tunnel: w341 -> [w345]
                      tunnel: [w344] -> w336
                      tunnel: [w343] -> w335
                      tunnel: "Min" -> [w343]
                      tunnel: [w342] -> w333
                      tunnel: [w349] -> w338
                      tunnel: w336 -> [w349]
                      tunnel: w335 -> [w348]
                      tunnel: w333 -> [w346]
                      frame #0 {
                        n216 = call <userlib>:"CONEX-CC Get Negative Software Limit v2.vi"("Connection Cluster in"=w345) -> ("Left limit"=w342:dbl, "Connection Cluster out"=w344:T8)  [unwired: 9 in]
                      }
                      frame #1 {
                        n217 = Not Equal?(x=w348, y=w346) -> ()  [unwired: 1 out]
                        n218 = case shown="False" FALSE {
                          tunnel: w346 -> [w350 _]
                          frame False {
                            n219 = property on="Min" class="DigNum (strict)"("Value"=w350) -> ()  [unwired: 2 in, 2 out]
                            n220 = property on="Position History" class="WFChart (strict)"("YScale.Minimum"=w350) -> ()  [unwired: 2 in, 2 out]
                            n221 = property on="Position glissière" class="Slide (strict)"("Scale.Minimum"=w350) -> ()  [unwired: 2 in, 2 out]
                          }
                          frame True {
                            n222 = One Button Dialog(message="Set Min Error") -> ()  [unwired: 1 in, 1 out]
                          }
                        }
                      }
                    }
                  }
                  event "Set Max": Value Change {
                    n223 = event-data() -> ()  [unwired: 2 out]
                    n224 = property on="Set Max" class="Bool (strict)"("Value"=FALSE ("Set Max")) -> ()  [unwired: 2 in, 2 out]
                    n225 = call <userlib>:"CONEX-CC Set Positive Software Limit v2.vi"("Positive limit (right)"="Max", "Connection Cluster in"=w353) -> ("Connection Cluster out"=w357:T8)  [unwired: 9 in]
                    n226 = flat-sequence {
                      tunnel: w357 -> [w359]
                      tunnel: [w359] -> w354
                      tunnel: [w362] -> w352
                      tunnel: w354 -> [w360]
                      frame #0 {
                        n227 = Wait (ms)(milliseconds to wait=u32 600 ("attente (ms)")) -> ()  [unwired: 1 out]
                      }
                      frame #1 {
                        n228 = call <userlib>:"CONEX-CC Get Positive Software Limit v2.vi"("Connection Cluster in"=w360) -> ("Right limit"=w361:dbl, "Connection Cluster out"=w362:T8)  [unwired: 9 in]
                        n229 = property on="Max" class="DigNum (strict)"("Value"=w361) -> ()  [unwired: 2 in, 2 out]
                        n230 = property on="Position History" class="WFChart (strict)"("YScale.Maximum"=w361) -> ()  [unwired: 2 in, 2 out]
                        n231 = property on="Position glissière" class="Slide (strict)"("Scale.Maximum"=w361) -> ()  [unwired: 2 in, 2 out]
                      }
                    }
                  }
                  event "Set velocity": Value Change {
                    n232 = event-data() -> ()  [unwired: 2 out]
                    n233 = flat-sequence {
                      tunnel: w366 -> [w368]
                      tunnel: [w367] -> w364
                      tunnel: [w371] -> w365
                      tunnel: w364 -> [w371]
                      tunnel: w365 -> [w375]
                      tunnel: [w374] -> w363
                      frame #0 {
                        n234 = call <userlib>:"CONEX-CC Set Velocity v2.vi"("Velocity"="Velocity:", "Connection Cluster in"=w368) -> ("Connection Cluster out"=w367:T8)  [unwired: 9 in]
                      }
                      frame #1 {
                        n235 = Wait (ms)(milliseconds to wait=u32 250 ("attente (ms)")) -> ()  [unwired: 1 out]
                      }
                      frame #2 {
                        n236 = call <userlib>:"CONEX-CC Get Velocity v2.vi"("Connection Cluster in"=w375) -> ("Velocity"=w373:dbl, "Connection Cluster out"=w374:T8)  [unwired: 8 in, 1 out]
                        n237 = property on="Velocity:" class="DigNum (strict)"("Value"=w373) -> ()  [unwired: 2 in, 2 out]
                        n238 = property on="Set velocity" class="Bool (strict)"("Value"=FALSE ("Set velocity")) -> ()  [unwired: 2 in, 2 out]
                      }
                    }
                  }
                  event "Position glissière": Mouse Up {
                    n239 = event-data() -> ()  [unwired: 2 out]
                    n240 = property on="Position glissière" class="Slide (strict)"() -> ("Value"=w379:cluster{dbl, dbl})  [unwired: 2 in, 2 out]
                    n241 = Unbundle(w379) -> (w376:dbl)  [unwired: 1 out]
                    "Target position" <- w376
                    n242 = call <userlib>:"CONEX-CC Absolute Move v2.vi"("Target position"=w376, "Connection Cluster in"=w378) -> ("Connection Cluster out"=w377:T8)  [unwired: 5 in, 2 out]
                  }
                  event "Action": Value Change {
                    n243 = event-data() -> ()  [unwired: 2 out]
                    n244 = property on="Action" class="Bool (strict)"() -> ("BoolText.Text"=w383:string)  [unwired: 2 in, 2 out]
                    n245 = case shown="\"HOME\"" w383 {
                      tunnel: w382 -> [w385 w387 w389 w395 w397]
                      tunnel: [w384 w387 w388 w394 w399] -> w381
                      frame "ENABLE" {
                        n246 = call <userlib>:"CONEX-CC Enter-Leave DISABLE State v2.vi"("Ready? (false=DISABLE true=READY)"=TRUE ("Flag (false=DISABLE true=READY)"), "Connection Cluster in"=w385) -> ("Connection Cluster out"=w384:T8)  [unwired: 7 in]
                      }
                      frame Default {
                      }
                      frame "HOME" {
                        n247 = flat-sequence {
                          tunnel: w389 -> [w392]
                          tunnel: [w391] -> w388
                          frame #0 {
                            n248 = One Button Dialog(message="The Stage will go to the 0 position. Check that the travel is clean!") -> ()  [unwired: 1 in, 1 out]
                          }
                          frame #1 {
                            n249 = call <userlib>:"CONEX-CC Home search v2.vi"("Connection Cluster in"=w392) -> ("Connection Cluster out"=w391:T8)  [unwired: 5 in, 3 out]
                          }
                        }
                      }
                      frame "DISABLE" {
                        n250 = call <userlib>:"CONEX-CC Enter-Leave DISABLE State v2.vi"("Ready? (false=DISABLE true=READY)"=FALSE ("Flag (false=DISABLE true=READY)"), "Connection Cluster in"=w395) -> ("Connection Cluster out"=w394:T8)  [unwired: 7 in]
                      }
                      frame "STOP" {
                        n251 = call <userlib>:"CONEX-CC Stop Motion v2.vi"("Connection Cluster in"=w397) -> ("Connection Cluster out"=w399:T8)  [unwired: 10 in]
                        n252 = property on="Stop cycle" class="Bool (strict)"("Value"=TRUE) -> ()  [unwired: 2 in, 2 out]
                        "Stop cycle" <- TRUE ("Stop cycle")
                      }
                    }
                    n253 = property on="Action" class="Bool (strict)"("Value"=FALSE) -> ()  [unwired: 2 in, 2 out]
                  }
                  event "-": Value Change {
                    n254 = event-data() -> ()  [unwired: 2 out]
                    n255 = property on="-" class="Bool (strict)"("Value"=FALSE ("-")) -> ()  [unwired: 2 in, 2 out]
                    n256 = Negate(x="Step:") -> (-x=w404:dbl)
                    n257 = property on="Units" class="CmbBox"() -> ("Value"=w402:string)  [unwired: 2 in, 2 out]
                    n258 = case shown="\"lam\"" w402 {
                      tunnel: [w407 w408 w411 w414] -> w403
                      tunnel: w404 -> [w407 w409 w412 w418]
                      frame "mm", Default {
                      }
                      frame "um" {
                        n259 = Multiply(x=w409, y=0.001) -> (x*y=w408:dbl)
                      }
                      frame "nm" {
                        n260 = Multiply(x=w412, y=1e-06) -> (x*y=w411:dbl)
                      }
                      frame "lam" {
                        n261 = Divide(x=w418, y=1000000.0) -> (x/y=w416:dbl)
                        n262 = property on="lambda" class="DigNum (strict)"() -> ("Value"=w415:dbl)  [unwired: 2 in, 2 out]
                        n263 = Multiply(x=w416, y=w415) -> (x*y=w414:dbl)
                      }
                    }
                    n264 = call <userlib>:"CONEX-CC Relative Move v2.vi"("Relative displacement"=w403, "Connection Cluster in"=w401) -> ("Connection Cluster out"=w400:T8)  [unwired: 9 in]
                  }
                  event "+": Value Change {
                    n265 = event-data() -> ()  [unwired: 2 out]
                    n266 = property on="+" class="Bool (strict)"("Value"=FALSE ("+")) -> ()  [unwired: 2 in, 2 out]
                    n267 = property on="Step:" class="DigNum (strict)"() -> ("Value"=w421:dbl)  [unwired: 2 in, 2 out]
                    n268 = property on="Units" class="CmbBox"() -> ("Value"=w420:string)  [unwired: 2 in, 2 out]
                    n269 = case shown="\"lam\"" w420 {
                      tunnel: [w425 w426 w429 w432] -> w419
                      tunnel: w421 -> [w425 w427 w430 w436]
                      frame "mm", Default {
                      }
                      frame "um" {
                        n270 = Multiply(x=w427, y=0.001) -> (x*y=w426:dbl)
                      }
                      frame "nm" {
                        n271 = Multiply(x=w430, y=1e-06) -> (x*y=w429:dbl)
                      }
                      frame "lam" {
                        n272 = Divide(x=w436, y=1000000.0) -> (x/y=w434:dbl)
                        n273 = property on="lambda" class="DigNum (strict)"() -> ("Value"=w433:dbl)  [unwired: 2 in, 2 out]
                        n274 = Multiply(x=w434, y=w433) -> (x*y=w432:dbl)
                      }
                    }
                    n275 = call <userlib>:"CONEX-CC Relative Move v2.vi"("Relative displacement"=w419, "Connection Cluster in"=w422) -> ("Connection Cluster out"=w423:T8)  [unwired: 9 in]
                  }
                  event "Go1": Value Change {
                    n276 = event-data() -> ()  [unwired: 2 out]
                    n277 = property on="Go1" class="Bool (strict)"("Value"=FALSE ("Go1")) -> ()  [unwired: 2 in, 2 out]
                    n278 = property on="Zero position" class="DigNum (strict)"() -> ("Value"=w440:dbl)  [unwired: 2 in, 2 out]
                    n279 = property on="Units" class="CmbBox"() -> ("Value"=w441:string)  [unwired: 2 in, 2 out]
                    n280 = Add(x="(1) Go to:", y=w440) -> (x+y=w438:dbl)
                    n281 = case shown="\"lam\"" w441 {
                      tunnel: [w445 w446 w449 w452] -> w437
                      tunnel: w438 -> [w445 w447 w450 w456]
                      frame "mm", Default {
                      }
                      frame "um" {
                        n282 = Multiply(x=w447, y=0.001) -> (x*y=w446:dbl)
                      }
                      frame "nm" {
                        n283 = Multiply(x=w450, y=1e-06) -> (x*y=w449:dbl)
                      }
                      frame "lam" {
                        n284 = Divide(x=w456, y=1000000.0) -> (x/y=w454:dbl)
                        n285 = property on="lambda" class="DigNum (strict)"() -> ("Value"=w453:dbl)  [unwired: 2 in, 2 out]
                        n286 = Multiply(x=w454, y=w453) -> (x*y=w452:dbl)
                      }
                    }
                    n287 = call <userlib>:"CONEX-CC Absolute Move v2.vi"("Target position"=w437, "Connection Cluster in"=w443) -> ("Connection Cluster out"=w442:T8)  [unwired: 5 in, 2 out]
                  }
                  event "Go2": Value Change {
                    n288 = event-data() -> ()  [unwired: 2 out]
                    n289 = property on="Go2" class="Bool (strict)"("Value"=FALSE ("Go2")) -> ()  [unwired: 2 in, 2 out]
                    n290 = property on="Zero position" class="DigNum (strict)"() -> ("Value"=w460:dbl)  [unwired: 2 in, 2 out]
                    n291 = property on="Units" class="CmbBox"() -> ("Value"=w461:string)  [unwired: 2 in, 2 out]
                    n292 = Add(x="(2) Go to:", y=w460) -> (x+y=w458:dbl)
                    n293 = case shown="\"lam\"" w461 {
                      tunnel: [w465 w467 w470 w473] -> w457
                      tunnel: w458 -> [w465 w466 w469 w472]
                      frame "mm", Default {
                      }
                      frame "um" {
                        n294 = Multiply(x=w466, y=0.001) -> (x*y=w467:dbl)
                      }
                      frame "nm" {
                        n295 = Multiply(x=w469, y=1e-06) -> (x*y=w470:dbl)
                      }
                      frame "lam" {
                        n296 = Divide(x=w472, y=1000000.0) -> (x/y=w475:dbl)
                        n297 = property on="lambda" class="DigNum (strict)"() -> ("Value"=w474:dbl)  [unwired: 2 in, 2 out]
                        n298 = Multiply(x=w475, y=w474) -> (x*y=w473:dbl)
                      }
                    }
                    n299 = call <userlib>:"CONEX-CC Absolute Move v2.vi"("Target position"=w457, "Connection Cluster in"=w463) -> ("Connection Cluster out"=w462:T8)  [unwired: 5 in, 2 out]
                  }
                  event "Go0": Value Change {
                    n300 = event-data() -> ()  [unwired: 2 out]
                    n301 = property on="Zero position" class="DigNum (strict)"() -> ("Value"=w477:dbl)  [unwired: 2 in, 2 out]
                    n302 = property on="Go0" class="Bool (strict)"("Value"=FALSE ("Go2")) -> ()  [unwired: 2 in, 2 out]
                    n303 = property on="Units" class="CmbBox"() -> ("Value"=w478:string)  [unwired: 2 in, 2 out]
                    n304 = case shown="\"lam\"" w478 {
                      tunnel: [w483 w485 w488 w491] -> w479
                      tunnel: w477 -> [w483 w484 w487 w490]
                      frame "mm", Default {
                      }
                      frame "um" {
                        n305 = Multiply(x=w484, y=0.001) -> (x*y=w485:dbl)
                      }
                      frame "nm" {
                        n306 = Multiply(x=w487, y=1e-06) -> (x*y=w488:dbl)
                      }
                      frame "lam" {
                        n307 = Divide(x=w490, y=1000000.0) -> (x/y=w493:dbl)
                        n308 = property on="lambda" class="DigNum (strict)"() -> ("Value"=w492:dbl)  [unwired: 2 in, 2 out]
                        n309 = Multiply(x=w493, y=w492) -> (x*y=w491:dbl)
                      }
                    }
                    n310 = call <userlib>:"CONEX-CC Absolute Move v2.vi"("Target position"=w479, "Connection Cluster in"=w480) -> ("Connection Cluster out"=w481:T8)  [unwired: 5 in, 2 out]
                  }
                  event "Tare": Value Change {
                    n311 = event-data() -> ()  [unwired: 2 out]
                    n312 = property on="Tare" class="Bool (strict)"("Value"=FALSE ("Tare")) -> ()  [unwired: 2 in, 2 out]
                    n313 = property on="Current position" class="DigNum (strict)"() -> ("Value"=w495:dbl)  [unwired: 2 in, 2 out]
                    n314 = property on="Zero position" class="DigNum (strict)"("Value"=w495) -> ()  [unwired: 2 in, 2 out]
                  }
                  event "Cycle": Value Change {
                    (unwired) 0 ("Numérique")
                    n315 = event-data() -> ()  [unwired: 2 out]
                    n316 = property on="Cycle" class="Bool (strict)"("Value"=TRUE ("Cycle")) -> ()  [unwired: 2 in, 2 out]
                  }
                  event "Holo:", "X position 1", "Y position", "Fine:", "Fine:", "X position", "Y position 1", "Xoffset1", "Yoffset1", "Y position 2", "Fine:", "Y position 2", "Yoffset1 2", "X position 2", "Fine: 3", "X position 3", "Xoffset1 2": Value Change {
                    w539 = ".bmp" ("string")
                    # "X"
                    # "Y"
                    n317 = event-data() -> ()  [unwired: 3 out]
                    n318 = property on="Holo:" class="DigNum (strict)"() -> ("Value"=w503:dbl)  [unwired: 2 in, 2 out]
                    n319 = Path To String(path=path "C:/Users/Lab541/Desktop/David_Maluenda MAIN FOLDER/System") -> (string=w536:string)
                    n320 = Number To Decimal String(number=w503, width (-)=i16 1) -> (decimal integer string=w535:string)
                    n321 = Read from Text File(file (use dialog)=path "C:/Users/Lab541/Desktop/David_Maluenda MAIN FOLDER/System/+scripts/design_kinds.txt") -> (text=w533:string)  [unwired: 3 in, 3 out]
                    n322 = Decrement(x=w503) -> (x-1=w532:dbl)
                    n323 = Pick Line(multi-line string=w533, line index=w532) -> (output string=→"String 4":string)  [unwired: 1 in]
                    n324 = Concatenate Strings(w536, "\\Holograms\\Hologram2_" ("string"), w535, w539) -> (w541:string)
                    n325 = Concatenate Strings(w536, "\\Holograms\\Hologram1_" ("string"), w535, w539) -> (w531:string)
                    n326 = String To Path(string=w541) -> (path=w508:path)
                    n327 = String To Path(string=w531) -> (path=w509:path)
                    n328 = case shown="1, Default" w503 {
                      tunnel: [w543 w544 path "C:/Users/Lab541/Desktop/David_Maluenda MAIN FOLDER/System/SupportFiles/Holos/SLM2_T100_ph0.png" ("Value") w547] -> w511
                      tunnel: [w543 w544 path "C:/Users/Lab541/Desktop/David_Maluenda MAIN FOLDER/System/SupportFiles/Holos/SLM1_T100_ph0.png" ("Value") w548] -> w510
                      tunnel: w509 -> [_ _ _ w548]
                      tunnel: w508 -> [_ _ _ w547]
                      frame 0 {
                        n329 = property on="test" class="Path"() -> ("Value"=w543:path)  [unwired: 2 in, 2 out]
                      }
                      frame -1 {
                        w544 = path "C:/Users/Lab541/Desktop/David_Maluenda MAIN FOLDER/System/SupportFiles/GrayLevel/0level.png" ("Value")
                      }
                      frame -2 {
                      }
                      frame 1, Default {
                      }
                    }
                    n330 = call "IMAQ ReadFile"("File Path"=w510, "Image"=w513) -> ("Image Out"=w502:T3)  [unwired: 5 in, 4 out]
                    n331 = call "IMAQ ReadFile"("File Path"=w511, "Image"=w512) -> ("Image Out"=w501:T3)  [unwired: 5 in, 4 out]
                    n332 = call "WinPositioner.vi"("Display?"=FALSE, "Yoffset 2"="Yoffset1 2", "Xoffset"="Xoffset1 2", "Image"=w501, "Y position"="Y position 2", "Fine Y position"="Fine:", "Fine X position"="Fine: 3", "X position"="X position 2") -> ("Y position"=→"Y position 2":dbl, "X position"=→"X position 3":dbl, "CGH_x"=→"CGHy":T3)  [unwired: 1 in]
                    n333 = call "WinPositioner.vi"("Display?"=TRUE, "Yoffset 2"="Yoffset1", "Xoffset"="Xoffset1", "Image"=w502, "Y position"="Y position", "Fine Y position"="Fine:", "Fine X position"="Fine:", "X position"="X position 1") -> ("Y position"=→"Y position 1":dbl, "X position"=→"X position":dbl, "CGH_x"=→"CGHx":T3)  [unwired: 1 in]
                  }
                  event "Units": Value Change {
                    n334 = event-data() -> ("NewVal"=w555:string, "OldVal"=w554:string)  [unwired: 1 out]
                    n335 = property on="(1) Go to:" class="DigNum (strict)"("Caption.Text"=w555) -> ()  [unwired: 2 in, 2 out]
                    n336 = property on="(2) Go to:" class="DigNum (strict)"("Caption.Text"=w555) -> ()  [unwired: 2 in, 2 out]
                    n337 = property on="Step:" class="DigNum (strict)"("Caption.Text"=w555) -> ()  [unwired: 2 in, 2 out]
                    n338 = property on="Current position" class="DigNum (strict)"("Caption.Text"=w555) -> ()  [unwired: 2 in, 2 out]
                    n339 = property on="Relative position" class="DigNum (strict)"("Caption.Text"=w555) -> ()  [unwired: 2 in, 2 out]
                    n340 = property on="Zero position" class="DigNum (strict)"("Caption.Text"=w555) -> ()  [unwired: 2 in, 2 out]
                    n341 = case shown="\"lam\"" w554 {
                      tunnel: [1000000.0 ("y") 1000.0 ("y") 1.0 ("y") w560] -> w553
                      frame "mm", Default {
                      }
                      frame "um" {
                      }
                      frame "nm" {
                      }
                      frame "lam" {
                        n342 = property on="lambda" class="DigNum (strict)"() -> ("Value"=w560:dbl)  [unwired: 2 in, 2 out]
                      }
                    }
                    n343 = case shown="\"nm\"" w555 {
                      tunnel: [1000000.0 ("y") 1000.0 ("y") 1.0 ("y") w564] -> w552
                      frame "mm", Default {
                      }
                      frame "um" {
                      }
                      frame "nm" {
                      }
                      frame "lam" {
                        n344 = property on="lambda" class="DigNum (strict)"() -> ("Value"=w564:dbl)  [unwired: 2 in, 2 out]
                      }
                    }
                    n345 = property on="Zero position" class="DigNum (strict)"() -> ("Value"=w550:dbl)  [unwired: 2 in, 2 out]
                    n346 = Divide(x=w553, y=w552) -> (x/y=w551:dbl)
                    n347 = Multiply(x=w550, y=w551) -> (x*y=w549:dbl)
                    n348 = property on="Zero position" class="DigNum (strict)"("Value"=w549) -> ()  [unwired: 2 in, 2 out]
                  }
                }
              }
              n349 = node-c288(w102) -> ()  [unwired: 1 out]
              n350 = node-c288(w104) -> ()  [unwired: 1 out]
              n351 = Unbundle By Name(w99) -> ("VISA resource name"=w98:refnum<visa-resource-name>, "error"=w97:errorcluster)
            }
            frame #3 {
            }
          }
        }
      }
      n352 = call <userlib>:"_Close Communications.vi"("Instrument Channel"=w31) -> ()  [unwired: 14 in, 1 out]
      n353 = call <vilib>:"Simple Error Handler.vi"("error in (no error)"=w35) -> ()  [unwired: 1 in, 8 out]
      n354 = call <vilib>:"Simple Error Handler.vi"("error in (no error)"=w24) -> ()  [unwired: 1 in, 8 out]
      n355 = call <vilib>:"Simple Error Handler.vi"("error in (no error)"=w25) -> ()  [unwired: 1 in, 8 out]
    }
  }
